vi "Write Opened.vi"(10 "Opened":bool, 11 "Waveform Session in":refnum<class "Waveform Session.lvclass">) -> (3 "Waveform Session out":refnum<class "Waveform Session.lvclass">)   [LabVIEW 2020, in "NI_VS Custom Device Waveform API.lvlib" / "Waveform Session.lvclass"]
uses:
  Waveform Session.lvclass
  Waveform Session.lvclass/Waveform Session.ctl
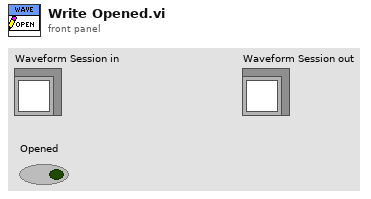
[diagram p1: front panel]
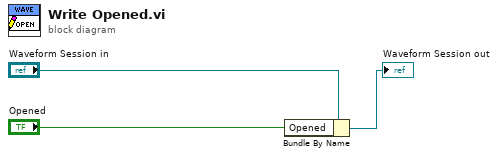
[diagram p0: block diagram]
diagram:
  n1 = Bundle By Name(cluster="Waveform Session in", "Opened"="Opened") -> (→"Waveform Session out":refnum<class "Waveform Session.lvclass">)
